vi "Read Unsigned Integer Configuration.vi"(7 "Type":T1, 8 "error in (no error)":errorcluster, 9 "Default If Not Found":u64, 10 "Name":string, 11 "IniFileSection in":refnum<class "IniFileSection.lvclass">) -> (0 "error out":errorcluster, 1 "Not Found?":bool, 2 "Value":u64, 3 "IniFileSection out":refnum<class "IniFileSection.lvclass">)   [LabVIEW 2017, in "IniFileSection.lvclass"]
uses:
  IniFileSection.lvclass
  <vilib>/Utility/Data Type/Type Definitions/Data Type.ctl
  IniFileSection.lvclass/IniFileSection.ctl
  <vilib>/Utility/error.llb/Error Cluster From Error Code.vi
  <vilib>/ErrorRing/Error Ring.xnode
  <vilib>/Utility/config.llb/NI_LVConfig.lvlib
  <vilib>/Utility/Data Type/NI_Data Type.lvlib
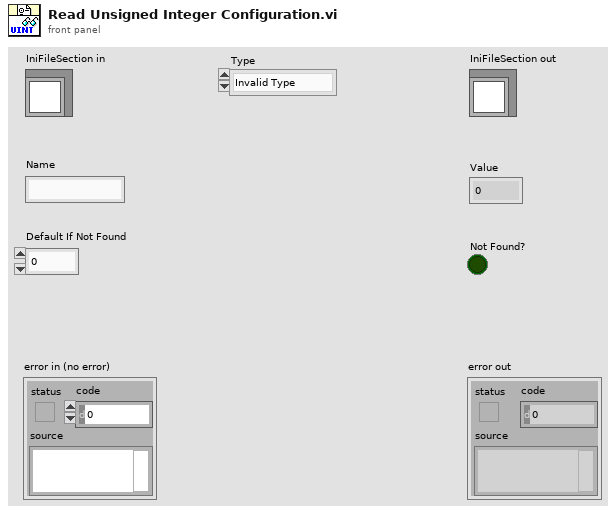
[diagram p1: front panel]
types:
  T1 = typedef "NI_Data Type.lvlib/Data Type.ctl" = enum8{"Invalid Type", "Void", "I8", "I16", "I32", "I64", "U8", "U16", "U32", "U64", "Single Float", "Double Float", "Extended Float", "Single Complex", "Double Complex", "Extended Complex", "Enum U8", "Enum U16", "Enum U32", "Enum U64", "Single Float With Unit", "Double Float With Unit", "Extended Float With Unit", "Single Complex with Unit", "Double Complex with Unit", "Extended Complex with Unit", "Boolean", "String", "Path", "Picture", "Tag", "Array", "Cluster", "Variant", "LV Variant", "Waveform", "Timestamp", "Digital Waveform", "Digital Data", "ExpressData", "Refnum", "External Data", "VI", "Poly VI", "LabVIEW Class Instance", "Fixed Point"}
  T2 = typedef "NI_LVConfig.lvlib/Config Data RefNum.ctl" = refnum<k1>
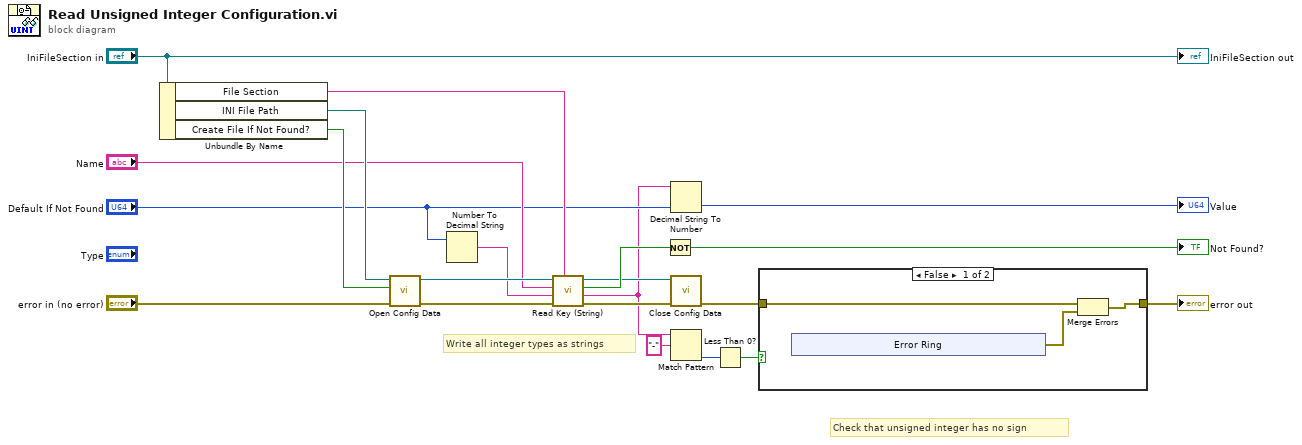
[diagram p0: block diagram]
diagram:
  # "Check that unsigned integer has no sign"
  # "Write all integer types as strings"
  n1 = Unbundle By Name("IniFileSection in") -> ("File Section"=w10:string, "INI File Path"=w18:path, "Create File If Not Found?"=w17:bool)
  n2 = call <vilib>:"Open Config Data.vi"("error in (no error)"="error in (no error)", "create file if necessary (T)"=w17, "configuration file path"=w18) -> ("error out"=w14:errorcluster, "refnum"=w21:T2)  [unwired: 6 in, 1 out]
  n3 = Number To Decimal String(number="Default If Not Found") -> (decimal integer string=w15:string)  [unwired: 1 in]
  n4 = call <vilib>:"Read Key (String).vi"("section"=w10, "error in (no error)"=w14, "default value"=w15, "key"="Name", "refnum"=w21) -> ("error out"=w13:errorcluster, "value"=w2:string, "found?"=w16:bool, "refnum out"=w12:T2)  [unwired: 3 in]
  n5 = Not(x=w16) -> (.not. x?=→"Not Found?":bool)
  n6 = Decimal String To Number(string=w2, default (0L)="Default If Not Found") -> (number=→"Value":u64)  [unwired: 1 in, 1 out]
  n7 = call <vilib>:"Close Config Data.vi"("error in (no error)"=w13, "refnum"=w12) -> ("error out"=w3:errorcluster)  [unwired: 8 in, 1 out]
  n8 = Match Pattern(string=w2, regular expression="-") -> (offset past match=w5:i32)  [unwired: 1 in, 3 out]
  n9 = Less Than 0?(x=w5) -> (x < 0?=w4:bool)
  n10 = case shown="False" w4 {
    tunnel: w3 -> [w24 w30]
    tunnel: [w23 w30] -> w1
    frame False {
      n11 = xnode "Error Ring"() -> ("error out"=w22:errorcluster)
      n12 = Merge Errors(w24, w22) -> (w23:errorcluster)
    }
    frame True {
      # "No \"-\" found, so no problem"
    }
  }
  "error out" <- w1
  "IniFileSection out" <- "IniFileSection in"
